vi "Analog Output Write.vi"(8 "error in":errorcluster, 10 "Analog Output Write":dbl[](array[numeric]) format="%0.2f", 11 "NI Analog Output in":refnum<class "NI Analog Output.lvclass">) -> (0 "error out":errorcluster, 3 "NI Analog Output out":refnum<class "NI Analog Output.lvclass">)   [LabVIEW 2023, in "HardwareAbstractionLayer_LVOOP.lvlib" / "NI Analog Output.lvclass"]
uses:
  NI Analog Output.lvclass
  NI Analog Output.lvclass/NI Analog Output.ctl
  <vilib>/DAQmx/write.llb/DAQmx Write (Analog 1D DBL NChan 1Samp).vi
  44c86652-e48f-4923-bb26-9afa66b7880d.vi
  <vilib>/DAQmx/miscellaneous.llb/DAQmx Fill In Error Info.vi
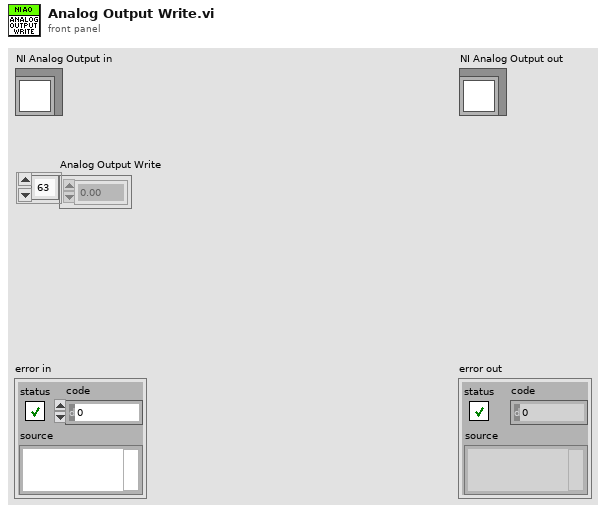
[diagram p1: front panel]
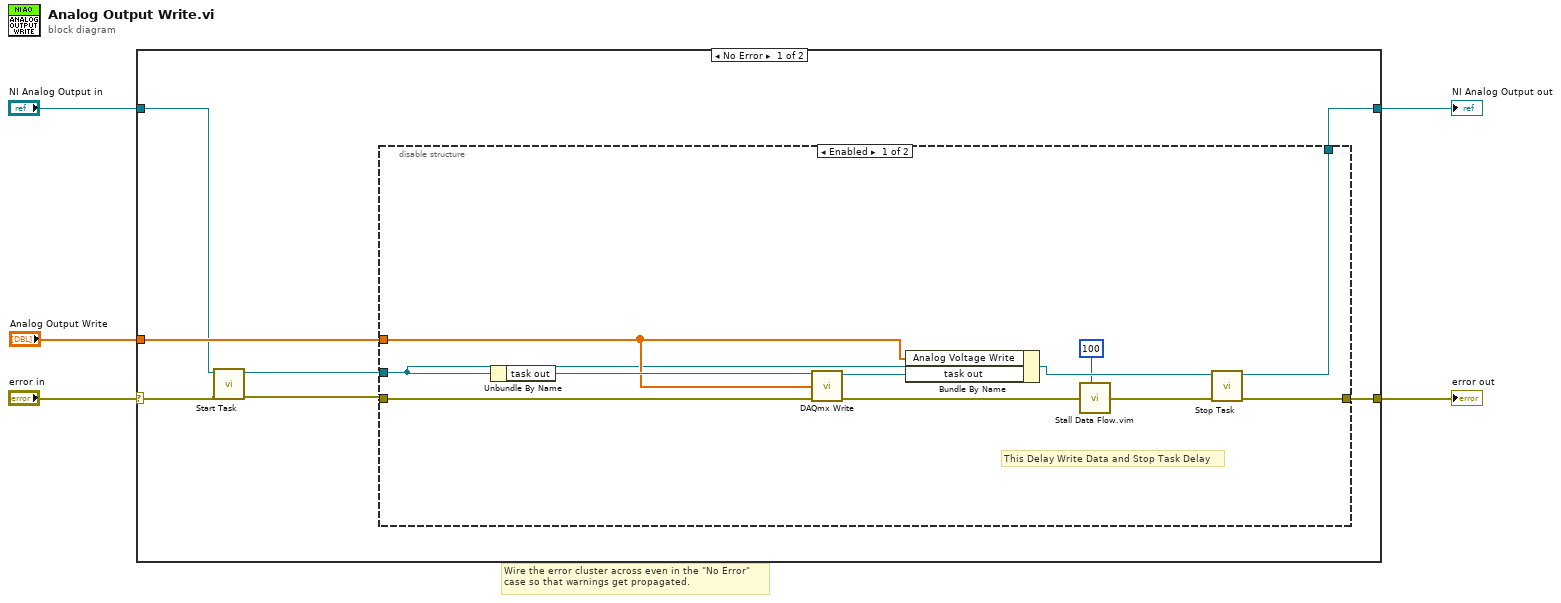
[diagram p0: block diagram]
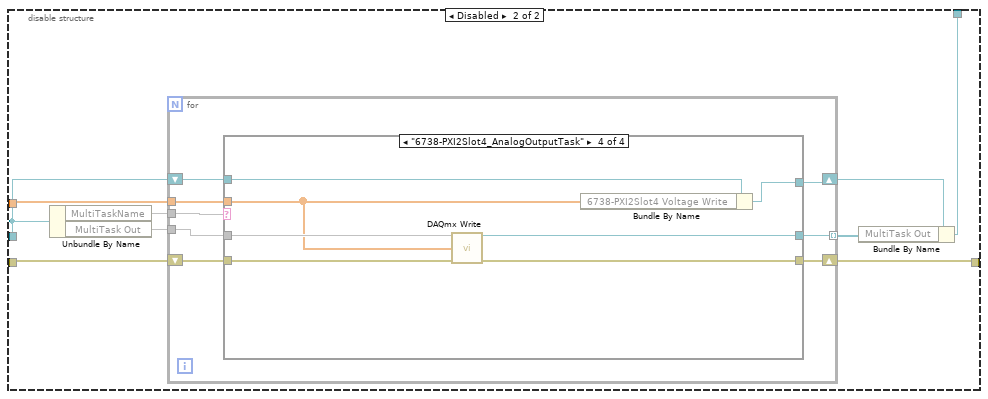
[diagram p2: hidden frame]
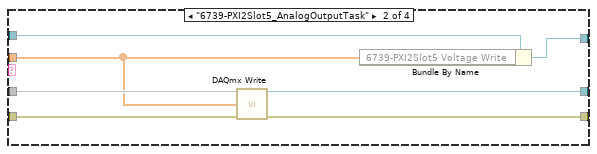
[diagram p4: hidden frame]
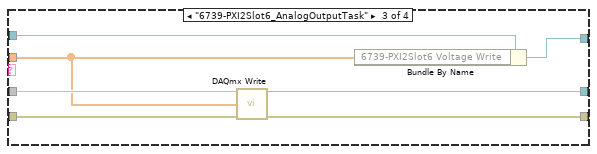
[diagram p5: hidden frame]
diagram:
  # "Wire the error cluster across even in the \"No Error\"\ncase so that warnings get propagated."
  n1 = case shown="No Error" "error in" {
    selector: "error in" -> [w8 w65]
    tunnel: [w12 w65] -> w4
    tunnel: [w11 w64] -> w2
    tunnel: "NI Analog Output in" -> [w9 w64]
    tunnel: "Analog Output Write" -> [w10 _]
    frame No Error {
      n2 = call-dynamic "Start Task.vi"("error in"=w8, "NI Analog Output in"=w9) -> ("error out"=w7:errorcluster, "NI Analog Output out"=w6:refnum<class "NI Analog Output.lvclass">)  [unwired: 8 in]
      n3 = disable-structure shown="Enabled" {
        disable-tunnel: w7 -> [w23 w32]
        disable-tunnel: [w15 w31] -> w12
        disable-tunnel: [w19 w27] -> _
        disable-tunnel: [w17 w25] -> w11
        disable-tunnel: w10 -> [w20 w30]
        disable-tunnel: w6 -> [w19 _]
        frame Enabled {
          # "This Delay Write Data and Stop Task Delay"
          n4 = Unbundle By Name(w19) -> ("task out"=w21:refnum<k21>)
          n5 = call-poly <vilib>:"DAQmx Write.vi"("task/channels in"=w21, "data"=w20, "error in"=w23) -> ("task out"=w22:refnum<k21>, "error out"=w16:errorcluster)  [unwired: 10 in, 1 out]
          n6 = Bundle By Name(cluster=w19, "Analog Voltage Write"=w20, "task out"=w22) -> (w18:refnum<class "NI Analog Output.lvclass">)
          n7 = call "Stall Data Flow.vim"("value in"=w16, "milliseconds to wait"=u32 100) -> ("value out"=w14:errorcluster)  [unwired: 1 out]
          n8 = call-dynamic "Stop Task.vi"("error in"=w14, "NI Analog Output in"=w18) -> ("error out"=w15:errorcluster, "NI Analog Output out"=w17:refnum<class "NI Analog Output.lvclass">)  [unwired: 8 in]
        }
        frame Disabled {
          n9 = Unbundle By Name(w27) -> ("MultiTaskName"=w29, "MultiTask Out"=w28)
          n10 = for {
            tunnel: w30 -> [w38]
            shift-right: [w39] -> w31
            shift-left: w32 -> [w40]
            tunnel: w29 -> [w37]
            tunnel: w28 -> [w36]
            shift-right: [w34] -> w26
            shift-left: w27 -> [w35]
            tunnel: [w33] -> w24 mode=indexing
            n11 = case shown="\"6738-PXI2Slot4_AnalogOutputTask\"" w37 {
              tunnel: w40 -> [w42 w49 w56 w63]
              tunnel: [w42 w48 w55 w62] -> w39
              tunnel: w38 -> [_ w43 w50 w57]
              tunnel: w36 -> [_ w47 w54 w61]
              tunnel: w35 -> [w41 w46 w53 w60]
              tunnel: [w41 w45 w52 w59] -> w34
              tunnel: [_ w44 w51 w58] -> w33
              frame "", Default {
              }
              frame "6739-PXI2Slot5_AnalogOutputTask" {
                n12 = call-poly <vilib>:"DAQmx Write.vi"("task/channels in"=w47, "data"=w43, "error in"=w49) -> ("task out"=w44:refnum<k21>, "error out"=w48:errorcluster)  [unwired: 10 in, 1 out]
                n13 = Bundle By Name(cluster=w46, "6739-PXI2Slot5 Voltage Write"=w43) -> (w45:refnum<class "NI Analog Output.lvclass">)
              }
              frame "6739-PXI2Slot6_AnalogOutputTask" {
                n14 = call-poly <vilib>:"DAQmx Write.vi"("task/channels in"=w54, "data"=w50, "error in"=w56) -> ("task out"=w51:refnum<k21>, "error out"=w55:errorcluster)  [unwired: 10 in, 1 out]
                n15 = Bundle By Name(cluster=w53, "6739-PXI2Slot6 Voltage Write"=w50) -> (w52:refnum<class "NI Analog Output.lvclass">)
              }
              frame "6738-PXI2Slot4_AnalogOutputTask" {
                n16 = call-poly <vilib>:"DAQmx Write.vi"("task/channels in"=w61, "data"=w57, "error in"=w63) -> ("task out"=w58:refnum<k21>, "error out"=w62:errorcluster)  [unwired: 10 in, 1 out]
                n17 = Bundle By Name(cluster=w60, "6738-PXI2Slot4 Voltage Write"=w57) -> (w59:refnum<class "NI Analog Output.lvclass">)
              }
            }
          }
          n18 = Bundle By Name(cluster=w26, "MultiTask Out"=w24) -> (w25:refnum<class "NI Analog Output.lvclass">)
        }
      }
    }
    frame Error {
    }
  }
  "error out" <- w4
  "NI Analog Output out" <- w2
